vi "Init Hardware.vi"(8 "error in (no error)":errorcluster, 11 "Strain Digitizer in":refnum<class "Strain Digitizer.lvclass">) -> (0 "error out":errorcluster, 3 "Strain Digitizer out":refnum<class "Strain Digitizer.lvclass">)   [LabVIEW 2016, in "Strain Digitizer.lvclass"]
uses:
  Strain Digitizer.lvclass
  C:/github/NHMFL_Core/Libraries/Instruments/Pulse Driver/Pulse Driver.lvclass
  Strain Digitizer.lvclass/Strain Digitizer.ctl
  Pulse Driver/Pulse Driver.lvclass/Pulse Driver.ctl
  Read VISA resource name.vi
  Pulse Driver/Read Samples per channel.vi
  Strain/Micron Optics sm130/Micron Optics sm130.lvlib
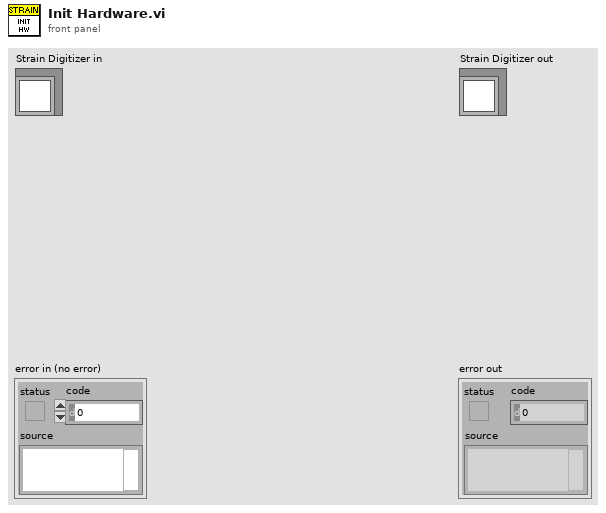
[diagram p1: front panel]
types:
  T1 = cluster{"Data Serial Number":u32, "Time Stamp":dbl, "Sub-Channel":u8}
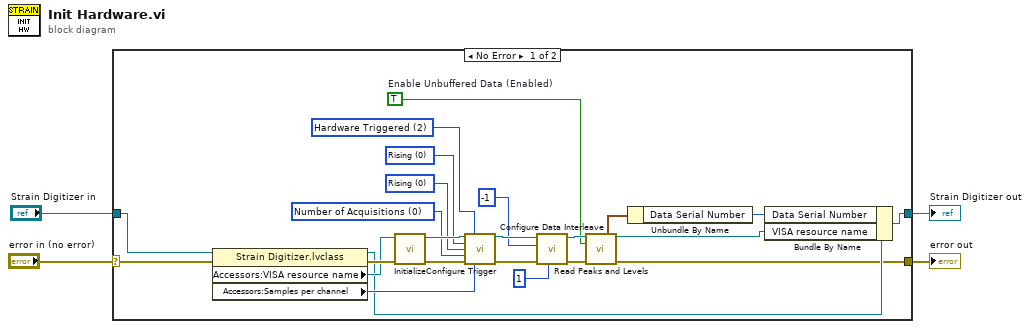
[diagram p0: block diagram]
diagram:
  n1 = case shown="No Error" "error in (no error)" {
    selector: "error in (no error)" -> [w23 w29]
    tunnel: "Strain Digitizer in" -> [w28 w30]
    tunnel: [w6 w30] -> w2
    tunnel: [w5 w29] -> w1
    frame No Error {
      w11 = TRUE  # Enable Unbuffered Data (Enabled)
      w18 = u16 0 items=["Number of Acquisitions", "Edge Triggering"] ("Trigger Stop Condition (1:Edge Triggering)")
      w19 = u16 0 items=["Rising", "Falling"] ("Trigger Stop Edge (0: Rising)")
      w20 = u16 0 items=["Rising", "Falling"] ("Trigger Start Edge (0: Rising)")
      w21 = u16 2 items=["Untriggered", "Software Triggered", "Hardware Triggered"] ("Trigger Type (0:Untriggered)")
      n2 = property class="Strain Digitizer.lvclass"(reference=w28, error in=w23) -> (reference out=w9:refnum<class "Strain Digitizer.lvclass">, error out=w27:errorcluster, "Accessors:VISA resource name"=w26:refnum<visa-resource-name>, "Accessors:Samples per channel"=w22:i32)
      n3 = call "Initialize.vi"("error in (no error)"=w27, "VISA resource name"=w26) -> ("error out"=w25:errorcluster, "VISA resource name out"=w24:refnum<visa-resource-name>)  [unwired: 8 in]
      n4 = call "Configure Trigger.vi"("VISA resource name"=w24, "Trigger Type (0:Untriggered)"=w21, "Trigger Start Edge (0: Rising)"=w20, "Trigger Stop Edge (0: Rising)"=w19, "Trigger Stop Condition (1:Edge Triggering)"=w18, "error in (no error)"=w25, "Number of Acquisitions (100)"=w22) -> ("VISA resource name out"=w17:refnum<visa-resource-name>, "error out"=w15:errorcluster)  [unwired: 6 in, 1 out]
      n5 = call "Configure Data Interleave.vi"("Data Interleave (1)"=1, "error in (no error)"=w15, "Sensor Number (1)"=-1, "VISA resource name"=w17) -> ("error out"=w12:errorcluster, "VISA resource name out"=w13:refnum<visa-resource-name>)  [unwired: 6 in]
      n6 = call "Read Peaks and Levels.vi"("VISA resource name"=w13, "Enable Unbuffered Data (Enabled)"=w11, "error in (no error)"=w12) -> ("Data Status"=w10:T1, "VISA resource name out"=w7:refnum<visa-resource-name>, "error out"=w5:errorcluster)  [unwired: 4 in, 6 out]
      n7 = Unbundle By Name(w10) -> ("Data Serial Number"=w8:u32)
      n8 = Bundle By Name(cluster=w9, "Data Serial Number"=w8, "VISA resource name"=w7) -> (w6:refnum<class "Strain Digitizer.lvclass">)
    }
    frame Error {
    }
  }
  "error out" <- w1
  "Strain Digitizer out" <- w2
